vi "testGetAllUserEventInstance.vi"(8 "error in (no error)":errorcluster) -> (0 "error out":errorcluster)   [LabVIEW 2018]
doc: "Test the getAllUserEventInstance.vi."
uses:
  src/TcpServer/TcpServer.lvclass
  src/TcpServer/typedef/userEventsTypeDef.ctl
  src/TcpServer/typedef/packetConnIDTypeDef.ctl
  src/TcpServer/typedef/ackTypeDef.ctl
  src/TcpServer/typedef/eventConnIDTypeDef.ctl
  <vilib>/addons/_JKI Toolkits/Caraya/classes/Assert/Assert Equal Type_Variant.vi
  <vilib>/addons/_JKI Toolkits/Caraya/classes/Test/Test.lvclass
  <vilib>/addons/_JKI Toolkits/Caraya/classes/Assert/Assert.lvclass
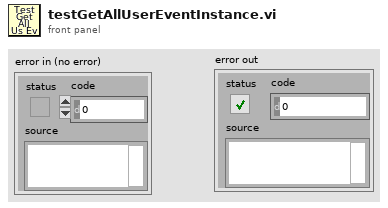
[diagram p1: front panel]
types:
  T1 = typedef "TcpServer.lvclass/userEventsTypeDef.ctl" = cluster{"TcpServer":refnum<user-event>, "Cmd":refnum<user-event>, "CmdStatus":refnum<user-event>, "Event":refnum<user-event>}
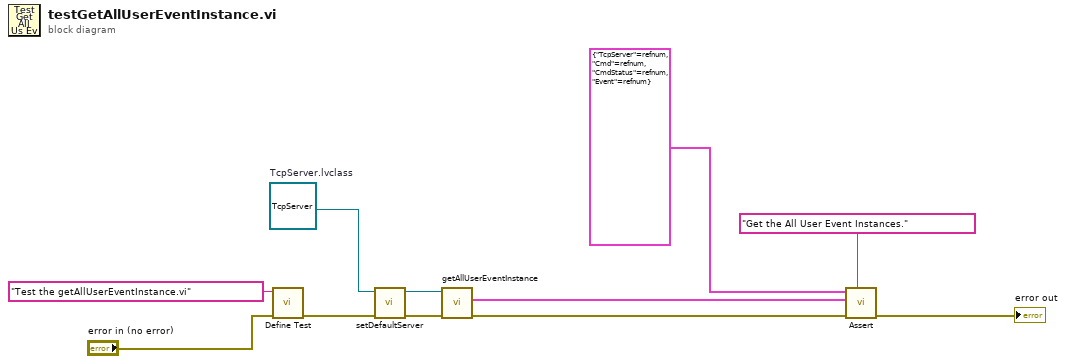
[diagram p0: block diagram]
diagram:
  w8 = refnum<class "TcpServer.lvclass"> refnum  # TcpServer.lvclass
  n1 = call <vilib>:"Define Test.vi"("error in (no error)"="error in (no error)", "Label (VI Title)"="Test the getAllUserEventInstance.vi") -> ("error out"=w10:errorcluster)  [unwired: 9 in]
  n2 = call "setDefaultServer.vi"("error in (no error)"=w10, "TcpServer.lvclass"=w8) -> ("error out"=w5:errorcluster, "tcpServer out"=w6:refnum<class "TcpServer.lvclass">)  [unwired: 8 in]
  n3 = call "getAllUserEventInstance.vi"("error in (no error)"=w5, "tcpServer in"=w6) -> ("error out"=w4:errorcluster, "UserEvents"=w1:T1)  [unwired: 7 in, 1 out]
  n4 = call-poly <vilib>:"Assert.vi"("Label"="Get the All User Event Instances.", "error in (no error)"=w4, "Y"=w1, "X"=T1 {"TcpServer"=refnum, "Cmd"=refnum, "CmdStatus"=refnum, "Event"=refnum} ("UserEvents")) -> ("error out"=→"error out":errorcluster)  [unwired: 7 in]
